vi "Compute SPARC.vi"(0 "Pressure Array":dbl[](array[numeric])=[1.0], 7 "Settings":string, 11 "error in":errorcluster) -> (4 "SPARC":dbl, 15 "error out":errorcluster)   [LabVIEW 2021]
uses:
  <vilib>/Analysis/NI_AALPro.lvlib
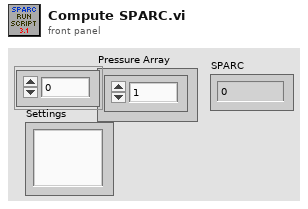
[diagram p1: front panel]
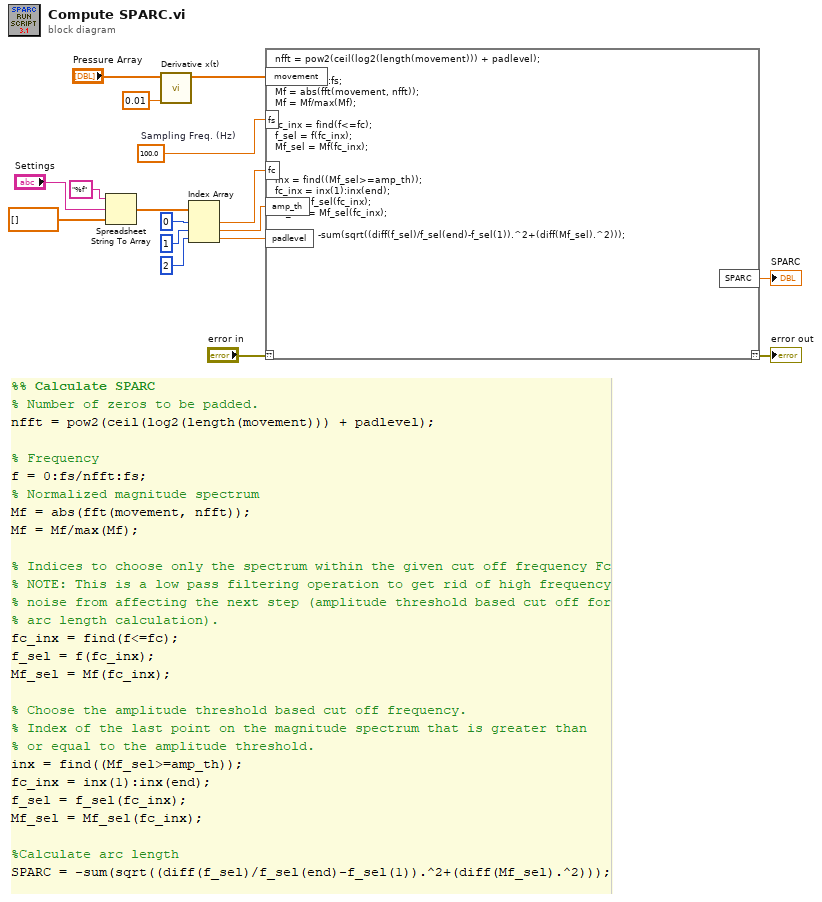
[diagram p0: block diagram]
diagram:
  w16 = 100.0  # Sampling Freq. (Hz)
  n1 = Spreadsheet String To Array(format string="%f", spreadsheet string="Settings", array type (2D Dbl)=dbl[] []) -> (array=w14:dbl[])  [unwired: 1 in]
  n2 = call <vilib>:"Derivative x(t).vi"("dt"=0.01, "X"="Pressure Array") -> ("dX/dt"=w3:dbl[])  [unwired: 8 in, 1 out]
  n3 = Index Array(array=w14, index #1=0 ("index"), index #2=1 ("index"), index #3=2 ("index")) -> (element #1=w9:dbl, element #2=w8:dbl, element #3=w7:dbl)
  n4 = script code="nfft = pow2(ceil(log2(length(movement))) + padlevel);\n\nf = 0:fs/nfft:fs;\nMf = abs(fft(movement, nfft));\nMf = Mf/max(Mf);\n\nfc_inx = find(f<=fc);\nf_sel = f(fc_inx);\nMf_sel = Mf(fc_inx);\n\n\ninx = find((Mf_sel>=amp_th));\nfc_inx = inx(1):inx(end);\nf_sel = f_sel(fc_inx);\nMf_sel = Mf_sel(fc_inx);\n\nSPARC = -sum(sqrt((diff(f_sel)/f_sel(end)-f_sel(1)).^2+(diff(Mf_sel).^2)));"("??"="error in", "movement"=w3, "fc"=w9, "padlevel"=w7, "amp_th"=w8, "fs"=w16) -> ("??"=→"error out":errorcluster, "SPARC"=→"SPARC":dbl)
